vi "VI-Delete Decorations.vi"(0 "VI in":refnum<vi>, 11 "error in (no error)":errorcluster) -> (4 "VI out":refnum<vi>, 15 "error out":errorcluster)   [LabVIEW 2020]
uses:
  <vilib>/Utility/traverseref.llb/TRef TravTarget.ctl
  <vilib>/Utility/traverseref.llb/VI Scripting - Traverse.lvlib
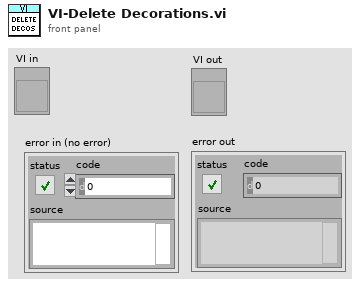
[diagram p1: front panel]
types:
  T1 = typedef "TRef TravTarget.ctl" = enum16{"FP", "BD", "Other"}
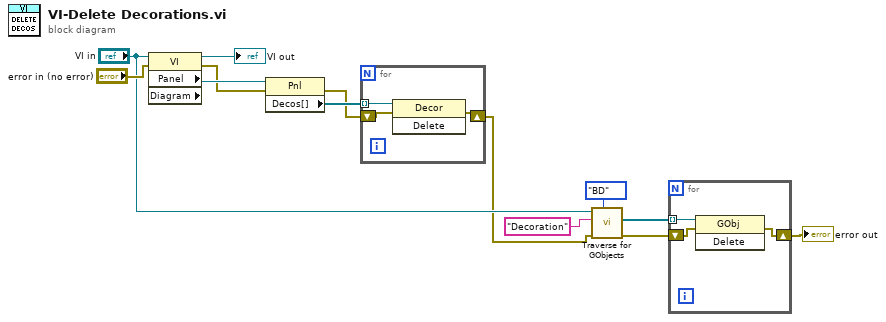
[diagram p0: block diagram]
diagram:
  n1 = property class="VI" props=["Panel", "Diagram"](reference="VI in", error in="error in (no error)") -> (reference out=→"VI out":refnum<vi>, error out=w10:errorcluster, "Panel"=w13:refnum<vi>)  [unwired: 1 out]
  n2 = property class="Pnl"(reference=w13, error in=w10) -> (error out=w9:errorcluster, "Decos[]"=w12:refnum<vi>[])  [unwired: 1 out]
  n3 = for {
    tunnel: w12 -> [w16] mode=indexing
    shift-right: [w14] -> w3
    shift-left: w9 -> [w15]
    n4 = invoke class="Decor" method="Delete"(reference=w16, error in=w15) -> (error out=w14:errorcluster)  [unwired: 1 in, 2 out]
  }
  n5 = call <vilib>:"Traverse for GObjects.vi"("Traverse Target"=TRef_TravTarget."BD", "error in (no error)"=w3, "Class Name"="Decoration", "VI Refnum"="VI in") -> ("error out"=w2:errorcluster, "References"=w5:refnum<vi>[])  [unwired: 4 in, 2 out]
  n6 = for {
    tunnel: w5 -> [w19] mode=indexing
    shift-right: [w17] -> w1
    shift-left: w2 -> [w18]
    n7 = invoke class="GObj" method="Delete"(reference=w19, error in=w18) -> (error out=w17:errorcluster)  [unwired: 1 in, 2 out]
  }
  "error out" <- w1
